vi "EOL CAN_Get Seed and Key.vi"(7 "Rx Arbitration Id":u32=402522244 format="%.0x", 8 "Error in":errorcluster, 10 "Read Session in":refnum<k21>, 11 "Write Session in":refnum<k21>) -> (0 "Error out":errorcluster, 2 "Response Good?":bool, 3 "TxRx Data":string[][](array[string]))   [LabVIEW 2014]
uses:
  <vilib>/xnet/xnet.llb/XNET Frame CAN.ctl
  <vilib>/xnet/xnet.llb/XNET Frame Type CAN.ctl
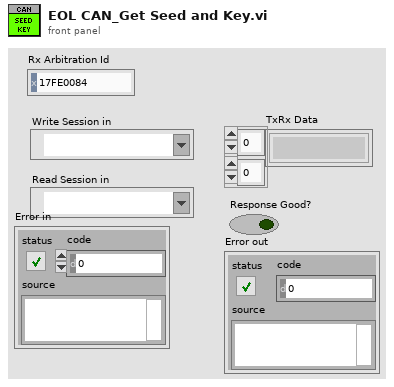
[diagram p1: front panel]
types:
  T1 = typedef "XNET Frame CAN.ctl" = cluster{"timestamp":timestamp, "payload":u8[], "identifier":u32, "type":T2, "extended?":bool, "echo?":bool}
  T2 = typedef "XNET Frame Type CAN.ctl" = u8
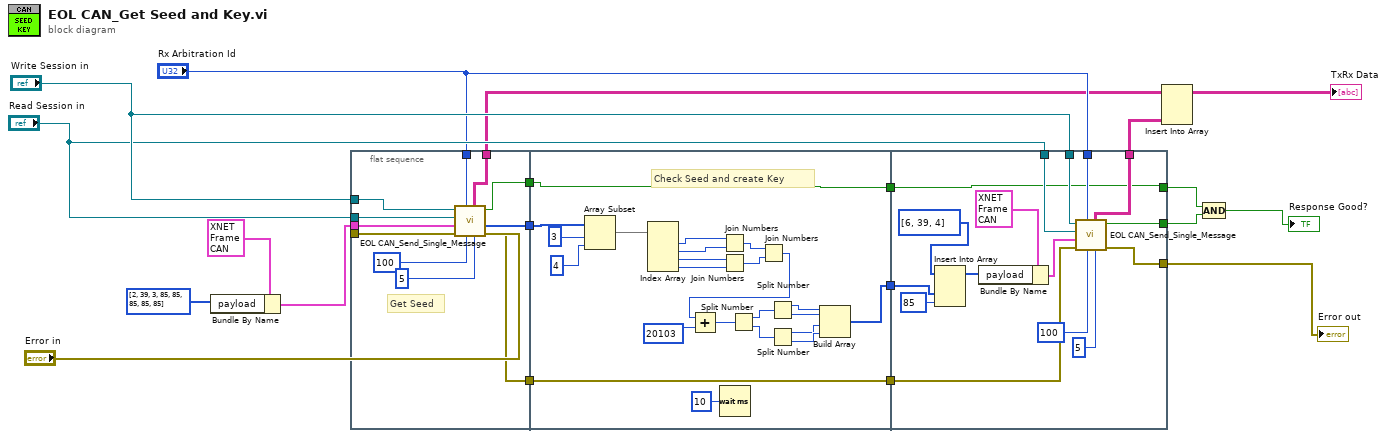
[diagram p0: block diagram]
diagram:
  n1 = Bundle By Name(cluster=T1 {"timestamp"=timestamp(0 s since 1904-01-01), "payload"=[2, 39, 3, 85, 85, 85, 85, 85], "identifier"=402391172, "type"=8, "extended?"=TRUE, "echo?"=FALSE} ("Tx CAN frame"), "payload"=u8[] [2, 39, 3, 85, 85, 85, 85, 85] ("Transmit Data 2")) -> (w18:T1)
  n2 = flat-sequence {
    tunnel: [w30] -> w8
    tunnel: w18 -> [w29]
    tunnel: "Read Session in" -> [w28]
    tunnel: "Write Session in" -> [w27]
    tunnel: "Error in" -> [w26]
    tunnel: "Rx Arbitration Id" -> [w24]
    tunnel: [w31] -> w16
    tunnel: [w25] -> w15
    tunnel: [w23] -> w13
    tunnel: w16 -> [w50]
    tunnel: w15 -> [w54]
    tunnel: [w54] -> w14
    tunnel: w13 -> [w53]
    tunnel: [w32] -> w12
    tunnel: [w50] -> w5
    tunnel: w14 -> [w70]
    tunnel: w12 -> [w62]
    tunnel: "Write Session in" -> [w67]
    tunnel: "Read Session in" -> [w66]
    tunnel: "Rx Arbitration Id" -> [w65]
    tunnel: [w64] -> w7
    tunnel: [w59] -> w2
    tunnel: w5 -> [w58]
    tunnel: [w58] -> w3
    tunnel: [w57] -> w1
    frame #0 {
      # "Get Seed"
      n3 = call "EOL CAN_Send_Single_Message.vi"("Retries"=5, "Msg Wait Time"=u32 100, "Rx Arbitration Id"=w24, "Error in"=w26, "Tx CAN frame"=w29, "Read Session in"=w28, "Write Session in"=w27) -> ("Error out"=w25:errorcluster, "Rx Message"=w23:u8[], "Response Good?"=w31:bool, "TxRx Data"=w30:string[][])  [unwired: 1 out]
    }
    frame #1 {
      # "Check Seed and create Key"
      n4 = Array Subset(array=w53, index=3, length=4) -> (w33:u8[])
      n5 = Index Array(array=w33) -> (element #1=w35:u8, element #2=w36:u8, element #3=w37:u8, element #4=w38:u8)  [unwired: 4 in]
      n6 = Join Numbers(hi=w35, lo=w36) -> ((hi.lo)=w39:u16)
      n7 = Join Numbers(hi=w37, lo=w38) -> ((hi.lo)=w40:u16)
      n8 = Wait (ms)(milliseconds to wait=u32 10) -> ()  [unwired: 1 out]
      n9 = Join Numbers(hi=w39, lo=w40) -> ((hi.lo)=w41:u32)
      n10 = Add(x=w41, y=u32 20103) -> (x+y=w42:u32)
      n11 = Split Number(x=w42) -> (hi(x)=w43:u16, lo(x)=w44:u16)
      n12 = Split Number(x=w43) -> (hi(x)=w45:u8, lo(x)=w46:u8)
      n13 = Split Number(x=w44) -> (hi(x)=w47:u8, lo(x)=w48:u8)
      n14 = Build Array(w45, w46, w47, w48) -> (w32:u8[])
    }
    frame #2 {
      n15 = Insert Into Array(array=u8[] [6, 39, 4] ("payload"), new element #1=w62, new element #2=u8 85 ("new element/subarray")) -> (w60:u8[])  [unwired: 1 in]
      n16 = Bundle By Name(cluster=T1 {"timestamp"=timestamp(0 s since 1904-01-01), "payload"=[2, 39, 3, 85, 85, 85, 85, 85], "identifier"=402391172, "type"=8, "extended?"=TRUE, "echo?"=FALSE} ("Tx CAN frame"), "payload"=w60) -> (w68:T1)
      n17 = call "EOL CAN_Send_Single_Message.vi"("Retries"=5, "Msg Wait Time"=u32 100, "Rx Arbitration Id"=w65, "Error in"=w70, "Tx CAN frame"=w68, "Read Session in"=w66, "Write Session in"=w67) -> ("Error out"=w57:errorcluster, "Response Good?"=w59:bool, "TxRx Data"=w64:string[][])  [unwired: 2 out]
    }
  }
  n18 = Insert Into Array(array=w8, new element=w7) -> (→"TxRx Data":string[][])  [unwired: 2 in]
  n19 = Compound Arithmetic op=AND(w3, w2) -> (→"Response Good?":bool)
  "Error out" <- w1
